vi "RegisterForMessageSpecificType.vi"(8 "error in (no error)":errorcluster, 9 "Message Enqueuer":refnum<class "Message Enqueuer.lvclass">, 10 "Message":refnum<class "MailBoxMessage.lvclass">, 11 "MailboxManager in":refnum<class "MailboxManager.lvclass">) -> (0 "error out":errorcluster, 3 "MailboxManager out":refnum<class "MailboxManager.lvclass">)   [LabVIEW 2020, in "MailboxManager.lvlib" / "MailboxManager.lvclass"]
uses:
  MailboxManager.lvclass
  MailBoxMessage/MailBoxMessage.lvclass
  <vilib>/ActorFramework/Message Enqueuer/Message Enqueuer.lvclass
  MailboxManager.lvclass/MailboxManager.ctl
  <vilib>/Utility/miscctls.llb/LVMapReplaceAction.ctl
  9247a740-fb26-4a05-b64d-42b46194273d.vi
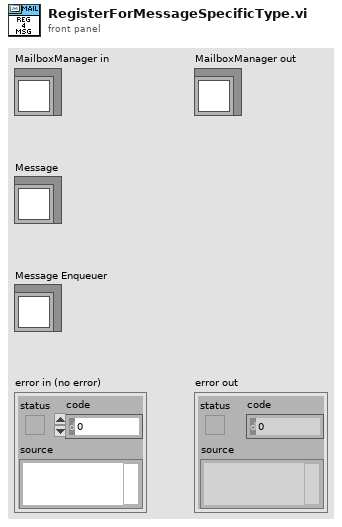
[diagram p1: front panel]
types:
  T1 = typedef "LVMapReplaceAction.ctl" = enum32{"Modify Entry only if found", "Add or Modify Entry", "Delete Entry"}
  T2 = map{refnum<class "MailBoxMessage.lvclass">, refnum<class "Message Enqueuer.lvclass">[]}
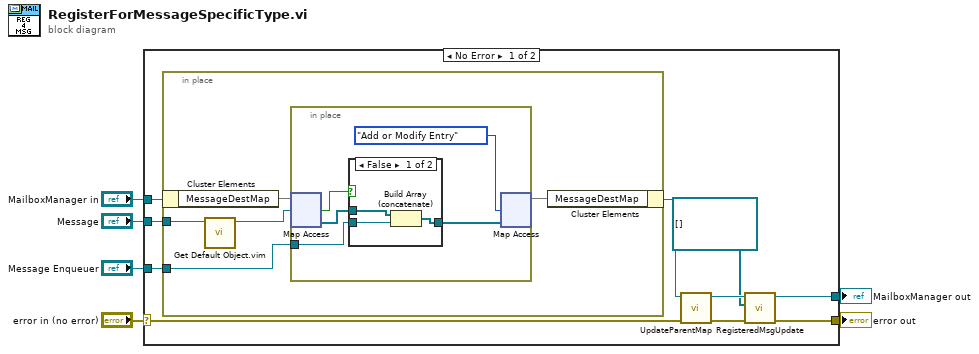
[diagram p0: block diagram]
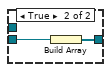
[diagram p2: hidden frame]
diagram:
  n1 = case shown="No Error" "error in (no error)" {
    selector: "error in (no error)" -> [w12 w33]
    tunnel: [w8 w33] -> w5
    tunnel: [w10 w32] -> w3
    tunnel: "MailboxManager in" -> [w16 w32]
    tunnel: "Message Enqueuer" -> [w14 _]
    tunnel: "Message" -> [w15 _]
    frame No Error {
      n2 = in-place {
        in-place-border: w15 -> [w18]
        in-place-border: w14 -> [w20]
        n3 = in-place-cluster #1(w16) -> ("MessageDestMap"=w21:T2)
        n4 = call "Get Default Object.vim"("MailBoxMessage in"=w18) -> ("MailBoxMessage out"=w17:refnum<class "MailBoxMessage.lvclass">)  [unwired: 10 in]
        n5 = in-place {
          in-place-border: w20 -> [w23]
          n6 = in-place-map #2(w21, w17) -> (w26:refnum<class "Message Enqueuer.lvclass">[], w24:bool)  [unwired: 1 in]
          n7 = case shown="False" w24 {
            tunnel: w26 -> [w29 _]
            tunnel: [w28 w30] -> w25
            tunnel: w23 -> [w27 w31]
            frame False {
              n8 = Build Array (concatenate)(w29, w27) -> (w28:refnum<class "Message Enqueuer.lvclass">[])
            }
            frame True {
              n9 = Build Array(w31) -> (w30:refnum<class "Message Enqueuer.lvclass">[])
            }
          }
          n10 = in-place-map #2(w25, LVMapReplaceAction."Add or Modify Entry" ("action")) -> (w19:T2)  [unwired: 2 out]
        }
        n11 = in-place-cluster #1("MessageDestMap"=w19) -> (w13:refnum<class "MailboxManager.lvclass">)
      }
      n12 = call "UpdateParentMap.vi"("error in (no error)"=w12, "MailboxManager in"=w13) -> ("error out"=w9:errorcluster, "MailboxManager out"=w11:refnum<class "MailboxManager.lvclass">)  [unwired: 8 in]
      n13 = call-dynamic "RegisteredMsgUpdate.vi"("error in (no error)"=w9, "Msgs"=refnum<class "MailBoxMessage.lvclass">[] [], "MailboxManager in"=w11) -> ("error out"=w8:errorcluster, "MailboxManager out"=w10:refnum<class "MailboxManager.lvclass">)  [unwired: 7 in]
    }
    frame Error {
    }
  }
  "error out" <- w5
  "MailboxManager out" <- w3
